vi "CRYDAT to Waveform.vi"(10 "dX":dbl, 11 "Curve In":T1={"Name"="", "Curve"=[], "X data"=1, "Y data"=1, "Z data"=1, "X axis"=0, "Y axis"=1, "Z axis"=1, "X unit"="Hz", "Y unit"="", "Z unit"="deg.", "X dB ref"=1.0, "Y dB ref"=1.0, "Z dB ref"=1.0, "single val"=FALSE, "protected"=FALSE, "display X"=TRUE, "display Y"=TRUE, "display Z"=TRUE, "Test Info"="", "Step No."=0, "Plot Settings"={"Color"=0, "Interpolation"=0, "Point Style"=0, "Line Style"=0, "Point Color"=0, "Line Width"=0, "Bar Plot Style"=0, "Fill To"=0}, "AutoProtect"=FALSE} {"Z data" items=["dB", "Lin"]; "X data" items=["dB", "Lin"]; "Y data" items=["dB", "Lin"]; "Z dB ref" format="%.1f"; "Z axis" items=["Log", "Lin"]; "X dB ref" format="%.1f"; "X axis" items=["Log", "Lin"]; "Y axis" items=["Log", "Lin"]; "Y dB ref" format="%.1f"; "Curve"."z" format="%.2f"; "Curve"."y" format="%.2f"; "Curve"."x" format="%.2f"}) -> (3 "Waveform Out":T2={"Waveform"={"X0"=0.0, "dX"=0.0, "Y"=[]}, "X data"=1, "Y data"=0, "Y axis"=0, "X unit"="s", "Y unit"="", "Y dB ref"=1.0, "display Y"=TRUE, "display X"=FALSE, "Overload?"=FALSE, "Test Info"="", "Step No."=0, "Name"="", "protected"=FALSE, "Sqc history"=[], "Signal Channel ID"=0, "Plot Settings"={"Color"=0, "Interpolation"=0, "Point Style"=0, "Line Style"=0, "Point Color"=0, "Line Width"=0, "Bar Plot Style"=0, "Fill To"=0}, "AutoProtect"=FALSE} {"Y dB ref" format="%.1f"; "Y axis" items=["Log", "Lin"]; "Y data" items=["dB", "Lin"]; "X data" items=["dB", "Lin"]})   [LabVIEW 2013]
uses:
  Typedef Control/CRYWaveform Cluster.ctl
  Typedef Control/CRYData Cluster.ctl
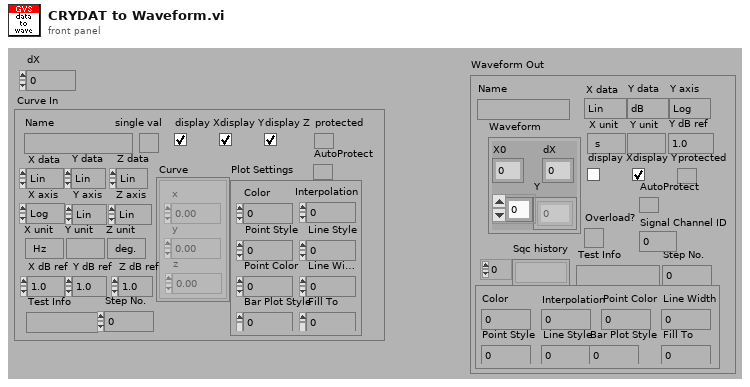
[diagram p1: front panel]
types:
  T1 = typedef "CRYData Cluster.ctl" = cluster{"Name":string, "Curve":cluster{"x":dbl, "y":dbl, "z":dbl}[], "X data":u16, "Y data":u16, "Z data":u16, "X axis":u16, "Y axis":u16, "Z axis":u16, "X unit":string, "Y unit":string, "Z unit":string, "X dB ref":dbl, "Y dB ref":dbl, "Z dB ref":dbl, "single val":bool, "protected":bool, "display X":bool, "display Y":bool, "display Z":bool, "Test Info":string, "Step No.":i32, "Plot Settings":cluster{"Color":u32, "Interpolation":u8, "Point Style":u8, "Line Style":u8, "Point Color":u32, "Line Width":u8, "Bar Plot Style":u8, "Fill To":i16}, "AutoProtect":bool}
  T2 = typedef "CRYWaveform Cluster.ctl" = cluster{"Waveform":cluster{"X0":dbl, "dX":dbl, "Y":sgl[]}, "X data":u16, "Y data":u16, "Y axis":u16, "X unit":string, "Y unit":string, "Y dB ref":dbl, "display Y":bool, "display X":bool, "Overload?":bool, "Test Info":string, "Step No.":i32, "Name":string, "protected":bool, "Sqc history":string[], "Signal Channel ID":i32, "Plot Settings":cluster{"Color":u32, "Interpolation":u8, "Point Style":u8, "Line Style":u8, "Point Color":u32, "Line Width":u8, "Bar Plot Style":u8, "Fill To":i16}, "AutoProtect":bool}
  T3 = cluster{"Color":u32, "Interpolation":u8, "Point Style":u8, "Line Style":u8, "Point Color":u32, "Line Width":u8, "Bar Plot Style":u8, "Fill To":i16}
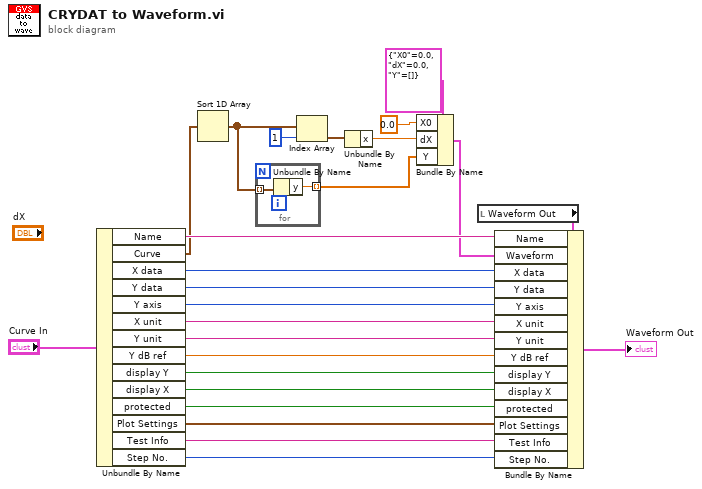
[diagram p0: block diagram]
diagram:
  n1 = Unbundle By Name("Curve In") -> ("Name"=w23:string, "Curve"=w8:cluster{"x":dbl, "y":dbl, "z":dbl}[], "X data"=w19:u16, "Y data"=w18:u16, "Y axis"=w17:u16, "X unit"=w16:string, "Y unit"=w15:string, "Y dB ref"=w14:dbl, "display Y"=w13:bool, "display X"=w12:bool, "protected"=w11:bool, "Plot Settings"=w10:T3, "Test Info"=w9:string, "Step No."=w7:i32)
  n2 = Sort 1D Array(array=w8) -> (sorted array=w2:cluster{"x":dbl, "y":dbl, "z":dbl}[])
  n3 = for {
    tunnel: w2 -> [w27] mode=indexing
    tunnel: [w26] -> w1 mode=indexing
    n4 = Unbundle By Name(w27) -> ("y"=w26:dbl)
  }
  n5 = Index Array(array=w2, index=1) -> (element=w4:cluster{"x":dbl, "y":dbl, "z":dbl})
  n6 = Unbundle By Name(w4) -> ("x"=w3:dbl)
  n7 = Bundle By Name(cluster=cluster{"X0":dbl, "dX":dbl, "Y":sgl[]} {"X0"=0.0, "dX"=0.0, "Y"=[]} ("Waveform"), "X0"=0.0, "dX"=w3, "Y"=w1) -> (w20:cluster{"X0":dbl, "dX":dbl, "Y":sgl[]})
  n8 = local read "Waveform Out"() -> (w24:T2)
  n9 = Bundle By Name(cluster=w24, "Name"=w23, "Waveform"=w20, "X data"=w19, "Y data"=w18, "Y axis"=w17, "X unit"=w16, "Y unit"=w15, "Y dB ref"=w14, "display Y"=w13, "display X"=w12, "protected"=w11, "Plot Settings"=w10, "Test Info"=w9, "Step No."=w7) -> (→"Waveform Out":T2)
